vi "Pulses.Count.vi"(8 "Dwell Limit":dbl, 9 "X 2":dbl, 10 "X":dbl, 11 "Waveform":waveform(dbl)) -> (3 "Numeric":i32)   [LabVIEW 2019, in "Fuel Injector Analysis Addon System Explorer.lvlib"]
uses:
  Fuel Injector Analysis Addon System Explorer.lvlib
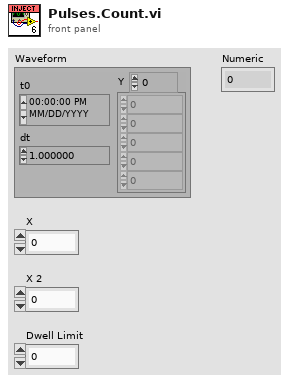
[diagram p1: front panel]
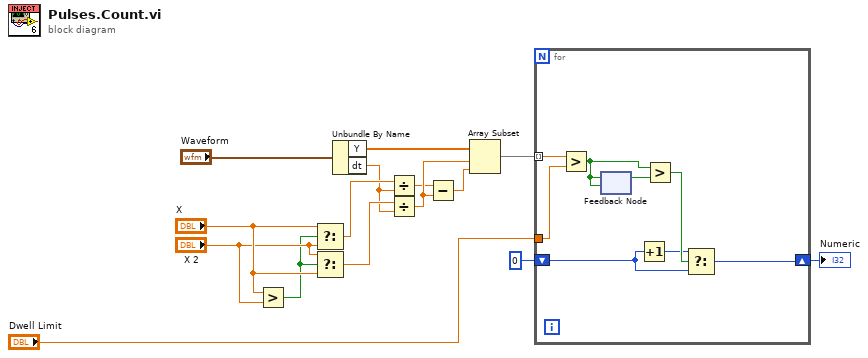
[diagram p0: block diagram]
diagram:
  n1 = Greater?(x="X", y="X 2") -> (0:w11:bool)
  n2 = Select(t="X", s=w11, f="X 2") -> (s? t:f=w14:dbl)
  n3 = Select(t="X 2", s=w11, f="X") -> (s? t:f=w15:dbl)
  n4 = Unbundle By Name("Waveform") -> ("Y"=w3:dbl[], "dt"=w6:dbl)
  n5 = Divide(x=w14, y=w6) -> (x/y=w2:dbl)
  n6 = Divide(x=w15, y=w6) -> (x/y=w4:dbl)
  n7 = Subtract(x=w2, y=w4) -> (x-y=w5:dbl)
  n8 = Array Subset(array=w3, index=w4, length=w5) -> (w8:dbl[])
  n9 = for {
    tunnel: "Dwell Limit" -> [w22]
    tunnel: w8 -> [w23] mode=indexing
    shift-right: [w20] -> w10
    shift-left: 0 -> [w19]
    n10 = Greater?(x=w23, y=w22) -> (0:w16:bool)
    n11 = feedback-in #1(w16) -> ()
    n12 = feedback #1(w16) -> (w17:bool)
    n13 = Increment(x=w19) -> (x+1=w18:i32)
    n14 = Greater?(x=w16, y=w17) -> (0:w21:bool)
    n15 = Select(t=w18, s=w21, f=w19) -> (s? t:f=w20:i32)
  }
  "Numeric" <- w10
